vi "rethinkdb_json_to_cluster.vi"(8 "error in (no error)":errorcluster, 11 "json":string) -> (0 "error out":errorcluster, 1 "invalid?":bool, 3 "cluster":variant)   [LabVIEW 2017]
uses:
  rethinkdb_json_token.ctl
  <vilib>/Utility/error.llb/Error Cluster From Error Code.vi
  <vilib>/ErrorRing/Error Ring.xnode
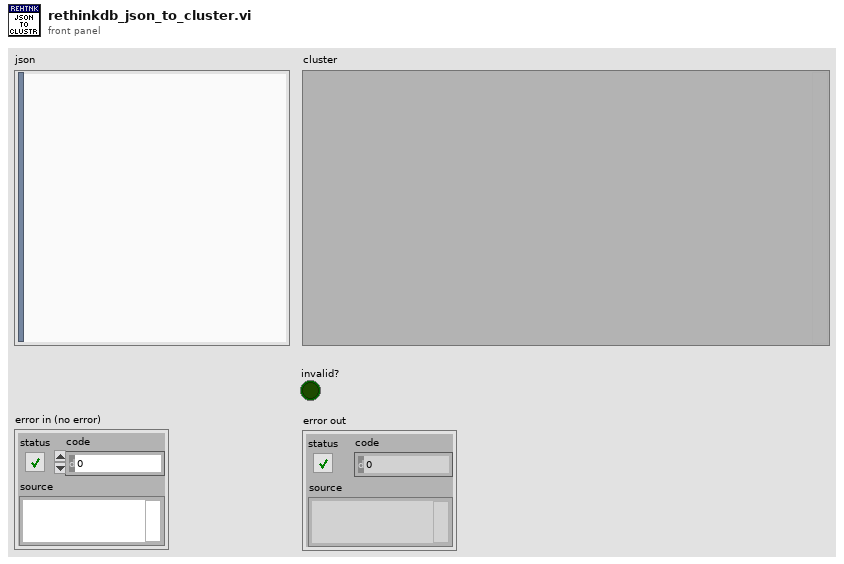
[diagram p1: front panel]
types:
  T1 = typedef "rethinkdb_json_token.ctl" = enum8{"invalid", "null", "boolean", "decimal", "float", "string", "key", "comma", "object_start", "object_end", "array_start", "array_end", "end"}
  T2 = cluster{"node":enum8{"object", "array"}, "values":variant[]}
  T3 = cluster{"node":enum8{"object", "array"}, "values":variant[]}[]
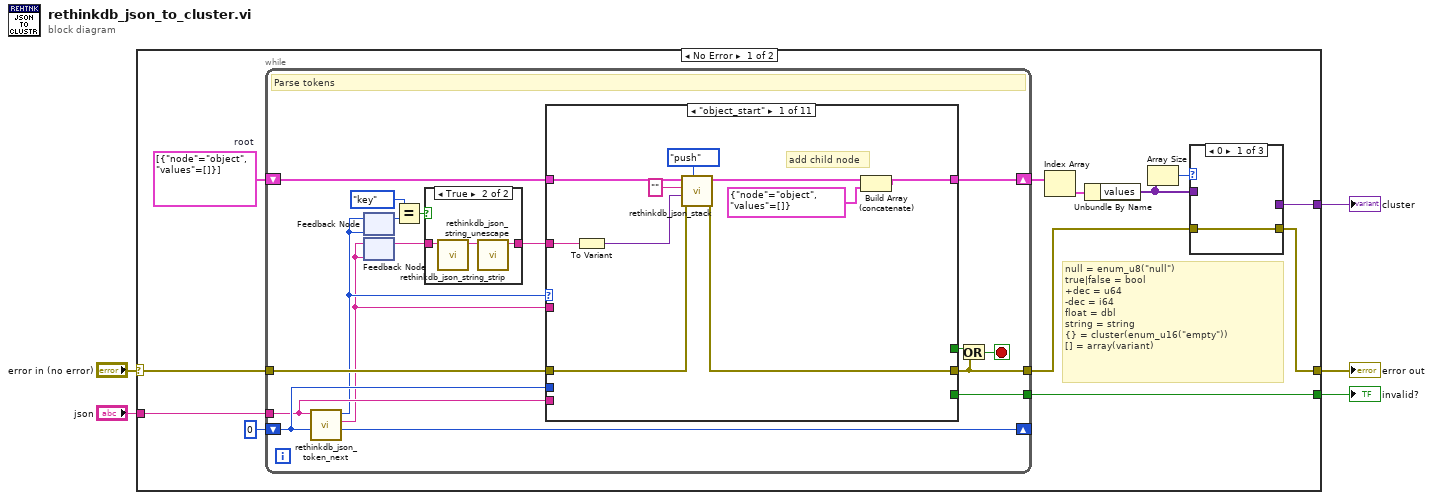
[diagram p0: block diagram]
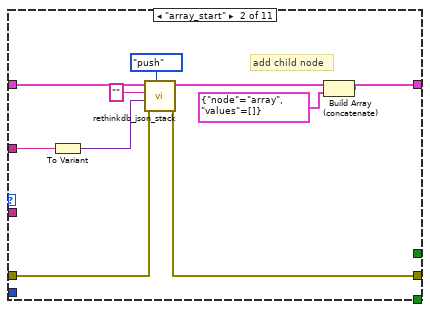
[diagram p3: hidden frame]
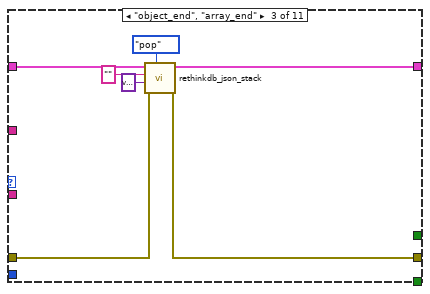
[diagram p4: hidden frame]
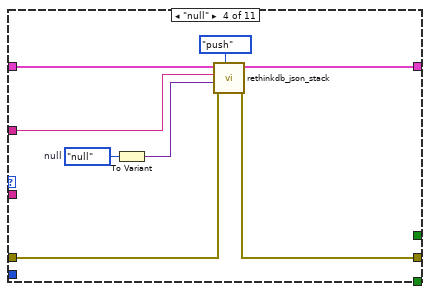
[diagram p5: hidden frame]
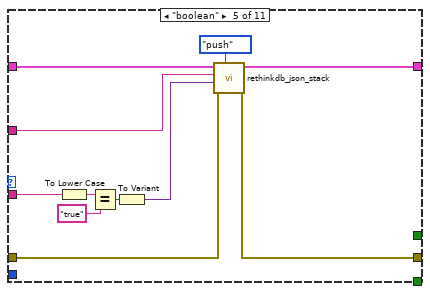
[diagram p6: hidden frame]
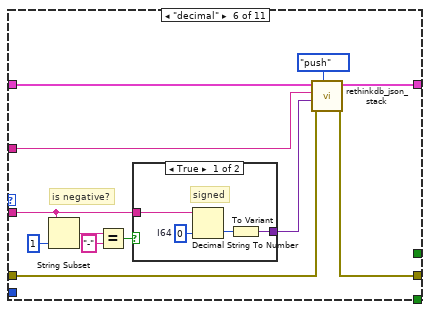
[diagram p7: hidden frame]
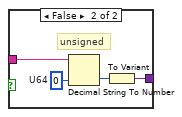
[diagram p8: hidden frame]
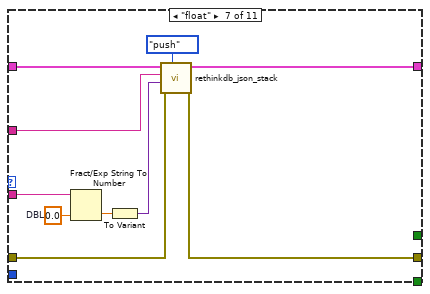
[diagram p9: hidden frame]
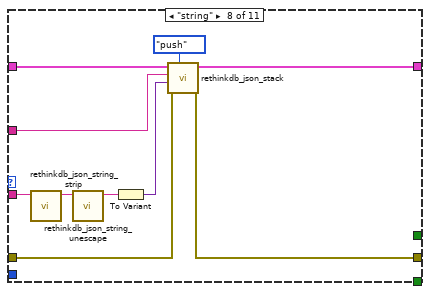
[diagram p10: hidden frame]
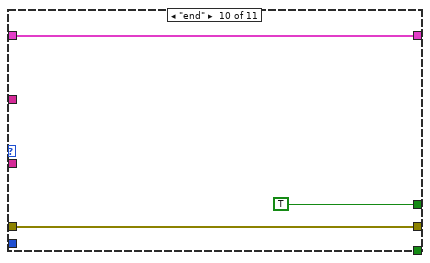
[diagram p12: hidden frame]
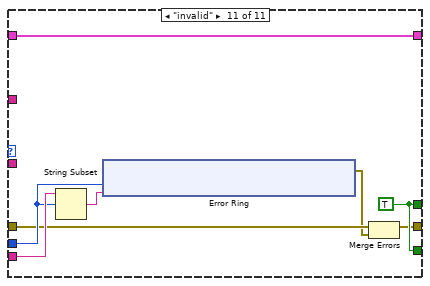
[diagram p13: hidden frame]
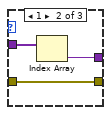
[diagram p14: hidden frame]
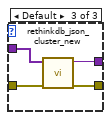
[diagram p15: hidden frame]
diagram:
  n1 = case shown="No Error" "error in (no error)" {
    selector: "error in (no error)" -> [w15 w153]
    tunnel: "json" -> [w17 _]
    tunnel: [w10 _] -> w3
    tunnel: [w8 w153] -> w2
    tunnel: [w7 _] -> w1
    frame No Error {
      w6 = T3 [{"node"=enum."object", "values"=[]}]  # root
      # "null = enum_u8(\"null\")\ntrue|false = bool\n+dec = u64\n-dec = i64\nfloat = dbl\nstring = string\n{} = cluster(enum_u16(\"empty\"))\n[] = array(variant)"
      n2 = while {
        tunnel: w17 -> [w31]
        shift-right: [w34] -> _
        shift-left: 0 ("offset past token") -> [w32]
        shift-right: [w26] -> w14
        shift-left: w6 -> [w21]
        tunnel: [w30] -> w9
        tunnel: w15 -> [w33]
        tunnel: [w28] -> w7
        stop <- w29 stop-if-true
        # "Parse tokens"
        n3 = call "rethinkdb_json_token_next.vi"("offset (0)"=w32, "json"=w31) -> ("offset past token"=w34:i32, "arg"=w22:string, "token"=w25:T1)  [unwired: 7 in]
        n4 = feedback-in #1(w25) -> ()
        n5 = feedback #1(w25) -> (w24:T1)
        n6 = feedback #2(w22) -> (w20:string)
        n7 = feedback-in #2(w22) -> ()
        n8 = Equal?(x=rethinkdb_json_token."key", y=w24) -> (x = y?=w18:bool)
        n9 = case shown="True" w18 {
          tunnel: w20 -> [_ w37]
          tunnel: [_ w35] -> w19
          frame False {
          }
          frame True {
            n10 = call "rethinkdb_json_string_strip.vi"("string in"=w37) -> ("string without first and last"=w36:string)  [unwired: 10 in]
            n11 = call "rethinkdb_json_string_unescape.vi"("escaped string"=w36) -> ("string out"=w35:string)  [unwired: 9 in, 1 out]
          }
        }
        n12 = case shown="\"object_start\"" w25 {
          tunnel: w33 -> [w41 w51 w61 w69 w80 w92 w110 w120 w124 w127 w131]
          tunnel: [w40 w50 w60 w68 w79 w91 w109 w119 w124 w127 w130] -> w30
          tunnel: w31 -> [_ _ _ _ _ _ _ _ _ _ w136]
          tunnel: w32 -> [_ _ _ _ _ _ _ _ _ _ w133]
          tunnel: w22 -> [_ _ _ _ w76 w85 w107 w115 _ _ _]
          tunnel: [_ _ _ _ _ _ _ _ _ _ w135] -> w28
          tunnel: [_ _ _ _ _ _ _ _ _ TRUE w135] -> w27
          tunnel: [w43 w53 w62 w70 w81 w93 w111 w121 w125 w128 w134] -> w26
          tunnel: w21 -> [w47 w57 w64 w72 w83 w95 w113 w123 w125 w128 w134]
          tunnel: w19 -> [w46 w56 _ w65 w77 w89 w108 w118 _ _ _]
          frame "object_start" {
            # "add child node"
            n13 = To Variant(anything=w46) -> (Variant=w39:variant)
            n14 = call "rethinkdb_json_stack.vi"("action"=enum8{"push", "pop"}."push", "error in (no error)"=w41, "value"=w39, "name"="", "stack in"=w47) -> ("error out"=w40:errorcluster, "stack out"=w45:T3)  [unwired: 5 in]
            n15 = Build Array (concatenate)(w45, T2 {"node"=enum."object", "values"=[]} ("object")) -> (w43:T3)
          }
          frame "array_start" {
            # "add child node"
            n16 = To Variant(anything=w56) -> (Variant=w49:variant)
            n17 = call "rethinkdb_json_stack.vi"("action"=enum8{"push", "pop"}."push", "error in (no error)"=w51, "value"=w49, "name"="", "stack in"=w57) -> ("error out"=w50:errorcluster, "stack out"=w55:T3)  [unwired: 5 in]
            n18 = Build Array (concatenate)(w55, T2 {"node"=enum."array", "values"=[]} ("object")) -> (w53:T3)
          }
          frame "object_end", "array_end" {
            n19 = call "rethinkdb_json_stack.vi"("action"=enum8{"push", "pop"}."pop", "error in (no error)"=w61, "value"=variant, "name"="", "stack in"=w64) -> ("error out"=w60:errorcluster, "stack out"=w62:T3)  [unwired: 5 in]
          }
          frame "null" {
            w67 = enum8{"null"}."null"  # null
            n20 = To Variant(anything=w67) -> (Variant=w66:variant)
            n21 = call "rethinkdb_json_stack.vi"("action"=enum8{"push", "pop"}."push", "error in (no error)"=w69, "value"=w66, "name"=w65, "stack in"=w72) -> ("error out"=w68:errorcluster, "stack out"=w70:T3)  [unwired: 5 in]
          }
          frame "boolean" {
            n22 = To Lower Case(string=w76) -> (all lower case string=w74:string)
            n23 = Equal?(x=w74, y="true") -> (x = y?=w75:bool)
            n24 = To Variant(anything=w75) -> (Variant=w78:variant)
            n25 = call "rethinkdb_json_stack.vi"("action"=enum8{"push", "pop"}."push", "error in (no error)"=w80, "value"=w78, "name"=w77, "stack in"=w83) -> ("error out"=w79:errorcluster, "stack out"=w81:T3)  [unwired: 5 in]
          }
          frame "decimal" {
            # "is negative?"
            n26 = String Subset(string=w85, length (rest)=1 ("length (rest)")) -> (substring=w87:string)  [unwired: 1 in]
            n27 = Equal?(x=w87, y="-") -> (x = y?=w84:bool)
            n28 = case shown="True" w84 {
              tunnel: [w99 w103] -> w90
              tunnel: w85 -> [w98 w102]
              frame True {
                w97 = i64 0  # I64
                # "signed"
                n29 = Decimal String To Number(string=w98, default (0L)=w97) -> (number=w96:i64)  [unwired: 1 in, 1 out]
                n30 = To Variant(anything=w96) -> (Variant=w99:variant)
              }
              frame False {
                w101 = u64 0  # U64
                # "unsigned"
                n31 = Decimal String To Number(string=w102, default (0L)=w101) -> (number=w100:u64)  [unwired: 1 in, 1 out]
                n32 = To Variant(anything=w100) -> (Variant=w103:variant)
              }
            }
            n33 = call "rethinkdb_json_stack.vi"("action"=enum8{"push", "pop"}."push", "error in (no error)"=w92, "value"=w90, "name"=w89, "stack in"=w95) -> ("error out"=w91:errorcluster, "stack out"=w93:T3)  [unwired: 5 in]
          }
          frame "float" {
            w106 = 0.0  # DBL
            n34 = Fract/Exp String To Number(string=w107, default (0 dbl)=w106) -> (number=w105:dbl)  [unwired: 2 in, 1 out]
            n35 = To Variant(anything=w105) -> (Variant=w104:variant)
            n36 = call "rethinkdb_json_stack.vi"("action"=enum8{"push", "pop"}."push", "error in (no error)"=w110, "value"=w104, "name"=w108, "stack in"=w113) -> ("error out"=w109:errorcluster, "stack out"=w111:T3)  [unwired: 5 in]
          }
          frame "string" {
            n37 = call "rethinkdb_json_string_strip.vi"("string in"=w115) -> ("string without first and last"=w114:string)  [unwired: 10 in]
            n38 = call "rethinkdb_json_string_unescape.vi"("escaped string"=w114) -> ("string out"=w117:string)  [unwired: 9 in, 1 out]
            n39 = To Variant(anything=w117) -> (Variant=w116:variant)
            n40 = call "rethinkdb_json_stack.vi"("action"=enum8{"push", "pop"}."push", "error in (no error)"=w120, "value"=w116, "name"=w118, "stack in"=w123) -> ("error out"=w119:errorcluster, "stack out"=w121:T3)  [unwired: 5 in]
          }
          frame "key", "comma" {
          }
          frame "end" {
          }
          frame "invalid" {
            w135 = TRUE
            n41 = String Subset(string=w136, offset (0)=w133) -> (substring=w132:string)  [unwired: 1 in]
            n42 = xnode "Error Ring"("parameter 0"=w133, "parameter 1"=w132) -> ("error out"=w129:errorcluster)
            n43 = Merge Errors(w131, w129) -> (w130:errorcluster)
          }
        }
        n44 = Or(x=w27, y=w30) -> (x .or. y?=w29:bool)
      }
      n45 = Index Array(array=w14) -> (element=w13:T2)  [unwired: 1 in]
      n46 = Unbundle By Name(w13) -> ("values"=w12:variant[])
      n47 = Array Size(array=w12) -> (size(s)=w11:i32)
      n48 = case shown="0" w11 {
        tunnel: w12 -> [_ w148 w152]
        tunnel: [_ w147 w151] -> w10
        tunnel: w9 -> [w145 w146 w150]
        tunnel: [w145 w146 w149] -> w8
        frame 0 {
        }
        frame 1 {
          n49 = Index Array(array=w148) -> (element=w147:variant)  [unwired: 1 in]
        }
        frame Default {
          n50 = call "rethinkdb_json_cluster_new.vi"("error in (no error)"=w150, "elements"=w152) -> ("error out"=w149:errorcluster, "cluster"=w151:variant)  [unwired: 8 in]
        }
      }
    }
    frame Error {
    }
  }
  "invalid?" <- w1
  "error out" <- w2
  "cluster" <- w3
